vi "System Semaphore Tree.vi"   [LabVIEW 2011]
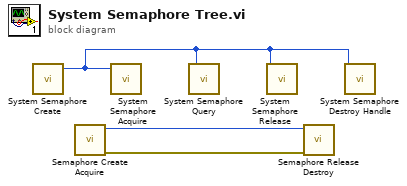
[diagram p0: block diagram]
diagram:
  n1 = call "System Semaphore Create.vi"() -> ("Handle"=w3:u16)  [unwired: 5 in, 1 out]
  n2 = call "Semaphore Create Acquire.vi"() -> ("error out"=w1:errorcluster, "TDM IO Lock"=w2:u16)  [unwired: 9 in, 1 out]
  n3 = call "System Semaphore Acquire.vi"("SemaphoreHandle"=w3) -> ()  [unwired: 2 in, 2 out]
  n4 = call "System Semaphore Query.vi"("SemaphoreHandle"=w3) -> ()  [unwired: 1 in, 4 out]
  n5 = call "System Semaphore Release.vi"("SemaphoreHandle"=w3) -> ()  [unwired: 2 in, 2 out]
  n6 = call "Semaphore Release Destroy.vi"("error in"=w1, "TDM IO Lock"=w2) -> ()  [unwired: 9 in, 1 out]
  n7 = call "System Semaphore Destroy Handle.vi"("SemaphoreHandle"=w3) -> ()  [unwired: 10 in, 1 out]
